vi "Two BTN Custom User Message.vi"(4 "Option 2 (\"Stop\")":string="Stop", 6 "Option 1 (\"OK\")":string="OK", 10 "Message":string) -> (1 "Ok?":bool)   [LabVIEW 2021]
panel:
  in  "Stop":bool
  in  "OK":bool
  in  "Title":string
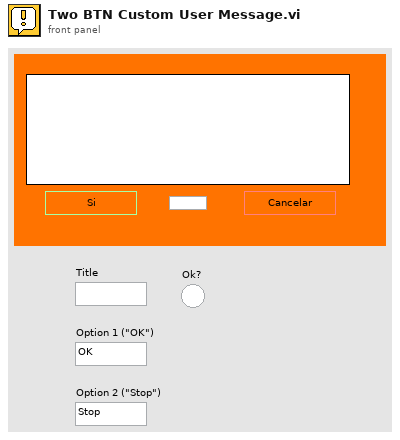
[diagram p1: front panel]
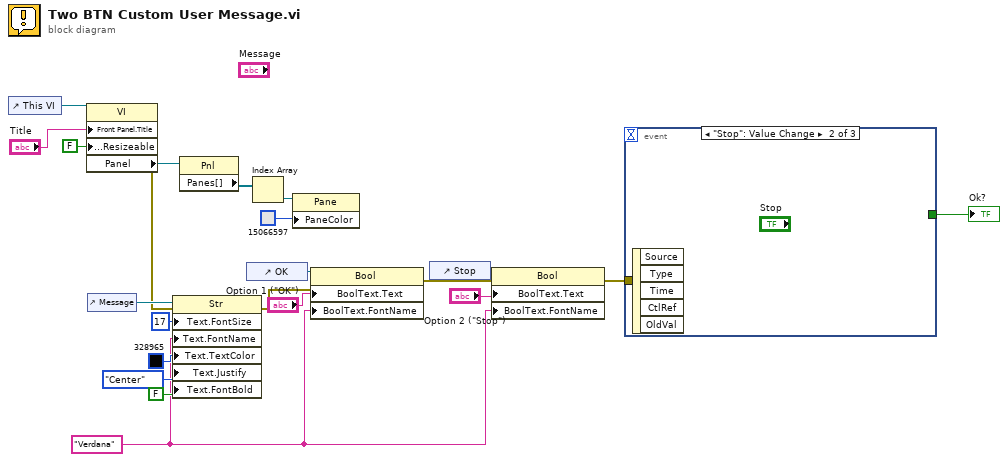
[diagram p0: block diagram]
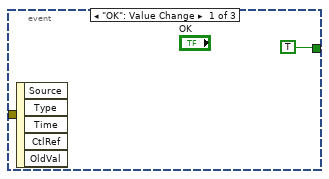
[diagram p2: hidden frame]
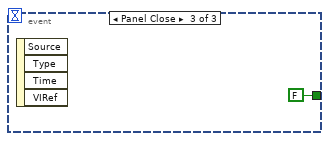
[diagram p3: hidden frame]
diagram:
  w1 = "Verdana" ("Text.Font:Name")
  n1 = control-ref of="This VI"() -> (w17:refnum<vi>)
  n2 = property class="VI"(reference=w17, "Front Panel.Title"="Title", "Front Panel.Resizeable"=FALSE ("Front Panel Window:Resizable")) -> (error out=w15:errorcluster, "Panel"=w13:refnum<vi>)  [unwired: 1 in, 1 out]
  n3 = control-ref of="Message"() -> (w22:refnum<vi>)
  n4 = property on="Property Node" class="Str"(reference=w22, error in=w15, "Text.FontSize"=u32 17 ("Text.Font:Size"), "Text.FontName"=w1, "Text.TextColor"=u32 328965 ("Text.Text Colors:Text Color"), "Text.Justify"=enum16{"Left", "Center", "Right"}."Center" ("Text.Justification"), "Text.FontBold"=FALSE ("Text.Font:Bold")) -> (error out=w7:errorcluster)  [unwired: 1 out]
  n5 = property class="Pnl"(reference=w13) -> ("Panes[]"=w12:refnum<vi>[])  [unwired: 1 in, 2 out]
  n6 = control-ref of="OK"() -> (w3:refnum<vi>)
  n7 = Index Array(array=w12) -> (element=w11:refnum<vi>)  [unwired: 1 in]
  n8 = property class="Pane"(reference=w11, "PaneColor"=u32 15066597 ("Pane Color")) -> ()  [unwired: 1 in, 2 out]
  n9 = property on="Property Node" class="Bool"(reference=w3, error in=w7, "BoolText.Text"="Option 1 (\"OK\")", "BoolText.FontName"=w1) -> (error out=w6:errorcluster)  [unwired: 1 out]
  n10 = control-ref of="Stop"() -> (w2:refnum<vi>)
  n11 = property on="Property Node" class="Bool"(reference=w2, error in=w6, "BoolText.Text"="Option 2 (\"Stop\")", "BoolText.FontName"=w1) -> (error out=w5:errorcluster)  [unwired: 1 out]
  n12 = event shown="[1] \"Stop\": Value Change" {
    selector: _ -> [_ _ _]
    dyn-events: _ -> [_ _ _]
    timeout: _ -> [_ _ _]
    tunnel: [TRUE _ FALSE] -> w18
    tunnel: w5 -> [_ _ _]
    event "OK": Value Change {
      n13 = event-data() -> ()  [unwired: 6 out]
    }
    event "Stop": Value Change {
      n14 = event-data() -> ()  [unwired: 6 out]
    }
    event Panel Close {
      n15 = event-data() -> ()  [unwired: 5 out]
    }
  }
  "Ok?" <- w18
